vi "Initialize Output Settings.vi"(8 "error in (no error)":errorcluster, 11 "Hardware Configuration":T1={"Task ID"=0, "Volume"=0.0, "Sample Rate"=0.0, "Duration"=0, "Data"={"SignalType"=enum."SineWave", "WhiteNoiseSettings"={"Generate New Data"=FALSE, "Save"=FALSE, "Filter"=TRUE, "Gain"=0.0}, "SineWaveSttings"={"Frequency"=0.0, "Amplitude"=0.0}}, "Generated Data"={"t0"=timestamp(0 s since 1904-01-01), "dt"=1.0, "Y"=[]}} {"task ID out" format="%.0x"}) -> (0 "error out":errorcluster, 3 "Hardware Configuration Out":T1={"Task ID"=0, "Volume"=0.0, "Sample Rate"=0.0, "Duration"=0, "Data"={"SignalType"=enum."SineWave", "WhiteNoiseSettings"={"Generate New Data"=FALSE, "Save"=FALSE, "Filter"=TRUE, "Gain"=0.0}, "SineWaveSttings"={"Frequency"=0.0, "Amplitude"=0.0}}, "Generated Data"={"t0"=timestamp(0 s since 1904-01-01), "dt"=1.0, "Y"=[]}} {"task ID out" format="%.0x"})   [LabVIEW 2022 SP3]
doc: "Initialize the hardware references."
uses:
  Output Hardware Configuration.ctl
  <vilib>/sound2/lvsound2.llb/Sound Output Task ID.ctl
  Data.ctl
  WhiteNoiseSettings.ctl
  SineWaveSettings.ctl
  <vilib>/sound2/lvsound2.llb/Sampling Mode.ctl
  <vilib>/sound2/lvsound2.llb/Sound Data Format.ctl
  <vilib>/sound2/lvsound2.llb/Sound Output Set Volume (Single).vi
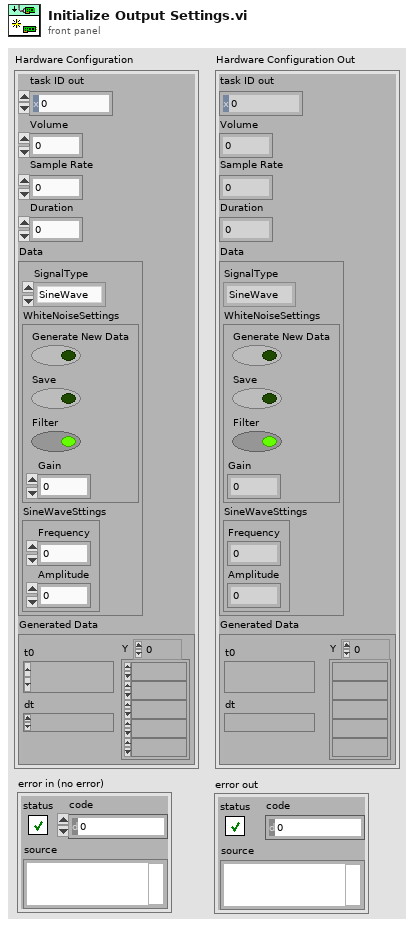
[diagram p1: front panel]
types:
  T1 = typedef "Output Hardware Configuration.ctl" = cluster{"Task ID":T2, "Volume":dbl, "Sample Rate":dbl, "Duration":i32, "Data":T3, "Generated Data":waveform(dbl)}
  T2 = typedef "Sound Output Task ID.ctl" = u32
  T3 = typedef "Data.ctl" = cluster{"SignalType":enum16{"WhiteNoise", "SineWave"}, "WhiteNoiseSettings":T4, "SineWaveSttings":T5}
  T4 = typedef "WhiteNoiseSettings.ctl" = cluster{"Generate New Data":bool, "Save":bool, "Filter":bool, "Gain":dbl}
  T5 = typedef "SineWaveSettings.ctl" = cluster{"Frequency":dbl, "Amplitude":dbl}
  T6 = typedef "Sound Data Format.ctl" = cluster{"sample rate (S/s)":dbl, "number of channels":i32, "bits per sample":i32}
  T7 = typedef "Sampling Mode.ctl" = i32
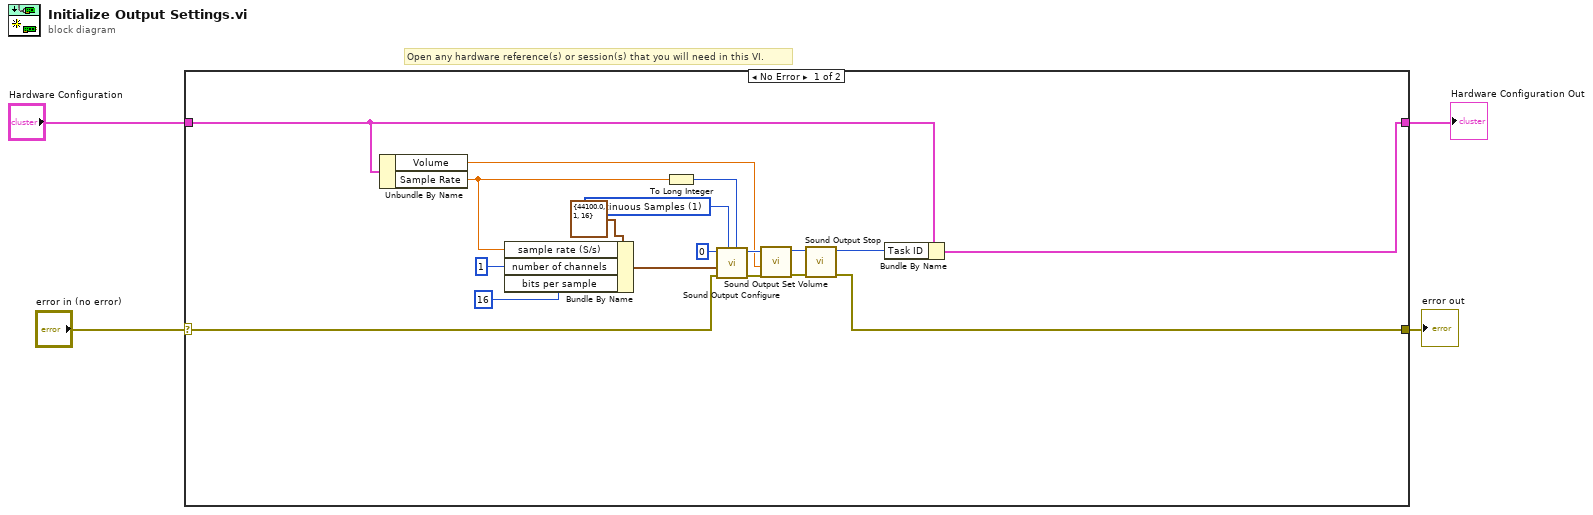
[diagram p0: block diagram]
diagram:
  # "Open any hardware reference(s) or session(s) that you will need in this VI."
  n1 = case shown="No Error" "error in (no error)" {
    selector: "error in (no error)" -> [w19 w23]
    tunnel: [w12 w23] -> w3
    tunnel: "Hardware Configuration" -> [w15 w24]
    tunnel: [w18 w24] -> w2
    frame No Error {
      w20 = T7 1 items=["Finite Samples", "Continuous Samples"] ("sample mode")
      n2 = Unbundle By Name(w15) -> ("Volume"=w16:dbl, "Sample Rate"=w10:dbl)
      n3 = Bundle By Name(cluster=T6 {"sample rate (S/s)"=44100.0, "number of channels"=1, "bits per sample"=16} ("Sound Format"), "sample rate (S/s)"=w10, "number of channels"=1, "bits per sample"=16) -> (w6:T6)
      n4 = To Long Integer(number=w10) -> (32bit integer=w5:i32)
      n5 = call <vilib>:"Sound Output Configure.vi"("number of samples/ch"=w5, "sample mode"=w20, "error in (no error)"=w19, "sound format"=w6, "device ID"=u32 0 ("Device ID")) -> ("error out"=w21:errorcluster, "task ID"=w22:T2)  [unwired: 5 in]
      n6 = call-poly <vilib>:"Sound Output Set Volume.vi"("error in (no error)"=w21, "volume"=w16, "task ID"=w22) -> ("error out"=w13:errorcluster, "task ID out"=w17:T2)  [unwired: 7 in]
      n7 = call <vilib>:"Sound Output Stop.vi"("error in (no error)"=w13, "task ID"=w17) -> ("error out"=w12:errorcluster, "task ID out"=w14:T2)  [unwired: 8 in]
      n8 = Bundle By Name(cluster=w15, "Task ID"=w14) -> (w18:T1)
    }
    frame Error {
    }
  }
  "error out" <- w3
  "Hardware Configuration Out" <- w2
